vi "Configure Preset.vi"(8 "error in (no error)":errorcluster, 10 "Preset":i32(ring) items=["Preset1", "Preset2", "Preset3", "Normal Mode"], 11 "VISA resource name":refnum<visa-resource-name>) -> (0 "error out":errorcluster, 3 "VISA resource name out":refnum<visa-resource-name>)   [LabVIEW 2022 SP3, in "BK Precision 9103.lvlib"]
doc: "Configures the preset value."
uses:
  <instrlib>/BK Precision 9103/BK Precision 9103.lvlib
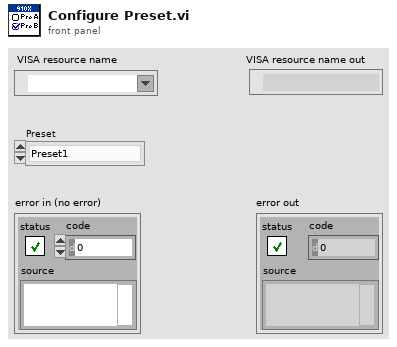
[diagram p1: front panel]
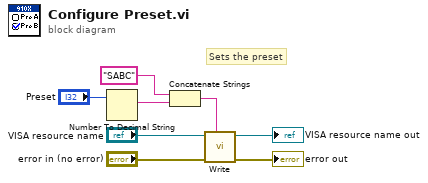
[diagram p0: block diagram]
diagram:
  # "Sets the preset"
  n1 = Number To Decimal String(number="Preset") -> (decimal integer string=w8:string)  [unwired: 1 in]
  n2 = Concatenate Strings("SABC" ("Send Command"), w8) -> (w5:string)
  n3 = call <instrlib>:"Write.vi"("Input String"=w5, "error in (no error)"="error in (no error)", "VISA resource name"="VISA resource name") -> ("error out"=→"error out":errorcluster, "VISA resource name out"=→"VISA resource name out":refnum<visa-resource-name>)  [unwired: 6 in, 1 out]
